vi "Set Active Sheet Namevi.vi"(8 "error in (no error)":errorcluster, 10 "Sheet Name":string, 11 "MS-Excel in":refnum<class "MS-Excel.lvclass">) -> (0 "error out":errorcluster, 3 "MS-Excel out":refnum<class "MS-Excel.lvclass">)   [LabVIEW 2017, in "LabVIEW NPOI.lvlib" / "MS-Excel.lvclass"]
uses:
  MS-Excel.lvclass
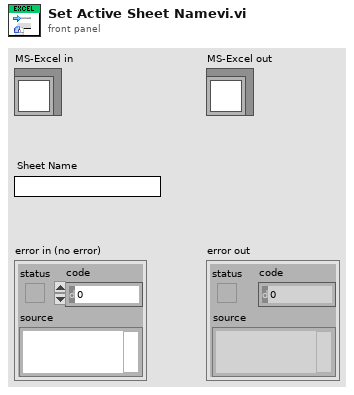
[diagram p1: front panel]
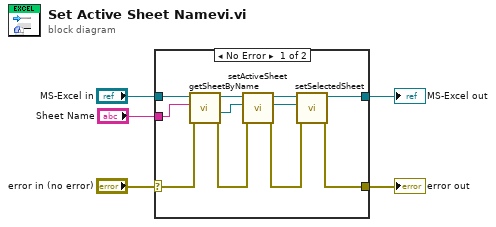
[diagram p0: block diagram]
diagram:
  n1 = case shown="No Error" "error in (no error)" {
    selector: "error in (no error)" -> [w7 w17]
    tunnel: [w12 w17] -> w4
    tunnel: [w14 w16] -> w2
    tunnel: "MS-Excel in" -> [w11 w16]
    tunnel: "Sheet Name" -> [w6 _]
    frame No Error {
      n2 = call-dynamic "getSheetByName.vi"("error in (no error)"=w7, "Sheet Name"=w6, "MS-Excel in"=w11) -> ("error out"=w8:errorcluster, "Sheet Ref"=w9:refnum<k24>, "MS-Excel out"=w10:refnum<class "MS-Excel.lvclass">)  [unwired: 5 in, 1 out]
      n3 = call-dynamic "setActiveSheet.vi"("error in (no error)"=w8, "Sheet Ref"=w9, "MS-Excel in"=w10) -> ("error out"=w13:errorcluster, "MS-Excel out"=w15:refnum<class "MS-Excel.lvclass">)  [unwired: 7 in]
      n4 = call-dynamic "setSelectedSheet.vi"("error in (no error)"=w13, "Sheet Ref"=w9, "MS-Excel in"=w15) -> ("error out"=w12:errorcluster, "MS-Excel out"=w14:refnum<class "MS-Excel.lvclass">)  [unwired: 7 in]
    }
    frame Error {
    }
  }
  "error out" <- w4
  "MS-Excel out" <- w2
